vi "ModifyGraph mirror.vi"(8 "error in (no error)":errorcluster, 10 "mirror [T]":bool=TRUE, 11 "ITX Commands in":refnum<class "ITX Commands.lvclass">) -> (0 "error out":errorcluster, 3 "ITX Commands out":refnum<class "ITX Commands.lvclass">)   [LabVIEW 2019, in "ITX Commands.lvclass"]
uses:
  ITX Commands.lvclass
  ITX Commands.lvclass/ITX Commands.ctl
panel:
  out "resulting string":string
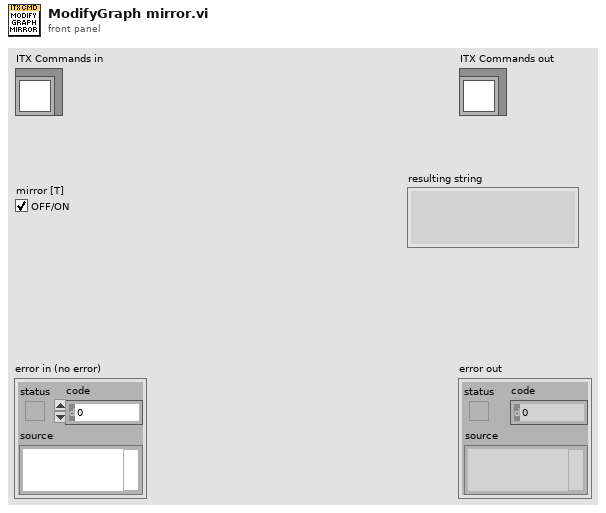
[diagram p1: front panel]
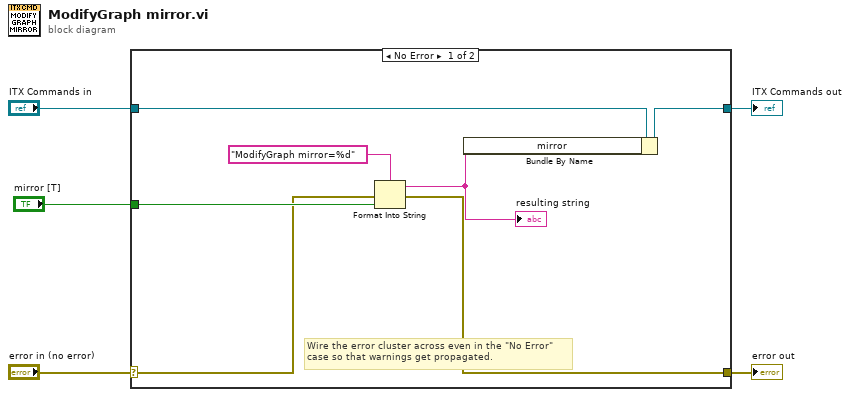
[diagram p0: block diagram]
diagram:
  n1 = case shown="No Error" "error in (no error)" {
    selector: "error in (no error)" -> [w7 w14]
    tunnel: [w6 w14] -> w4
    tunnel: [w11 w13] -> w2
    tunnel: "ITX Commands in" -> [w12 w13]
    tunnel: "mirror [T]" -> [w8 _]
    frame No Error {
      # "Wire the error cluster across even in the \"No Error\"\ncase so that warnings get propagated."
      n2 = Format Into String(format string="ModifyGraph mirror=%d", error in=w7, w8) -> (resulting string=w9:string, error out=w6:errorcluster)  [unwired: 1 in]
      "resulting string" <- w9
      n3 = Bundle By Name(cluster=w12, "mirror"=w9) -> (w11:refnum<class "ITX Commands.lvclass">)
    }
    frame Error {
    }
  }
  "error out" <- w4
  "ITX Commands out" <- w2
